vi "configureSerial.vi"(8 "error in (no error)":errorcluster, 10 "RS232Config":T1={"VISA resource name"="", "Baud Rate"=9600, "Data Bits"=8, "Parity"=enum."None", "Stop Bits"=10, "Flow Control"=0, "Timeout (ms)"=10000} {"Stop Bits" items=["1.0"=10, "1.5"=15, "2.0"=20]; "Flow Control" items=["None", "XON/XOFF", "RTS/CTS", "XON/XOFF & RTS/CTS", "DTR/DSR", "XON/XOFF & DTR/DSR"]; "Data Bits" min=5 max=8 step=1}, 11 "Model in":refnum<class "Model.lvclass">) -> (0 "error out":errorcluster, 3 "Model out":refnum<class "Model.lvclass">)   [LabVIEW 2012, in "Model.lvclass"]
uses:
  Model.lvclass
  Program Files (x86)/National Instruments/LabVIEW 2012/user.lib/Common/SerialProtocols/Configuration/RS232Config.ctl
  Program Files (x86)/National Instruments/LabVIEW 2012/user.lib/Common/SerialProtocols/Configuration/SerialProtocol.ctl
  Program Files (x86)/National Instruments/LabVIEW 2012/user.lib/Common/SerialProtocols/Implementations/SerialSimulator/SerialSimulator.lvclass
  Program Files (x86)/National Instruments/LabVIEW 2012/user.lib/Common/SerialProtocols/SerialCommunicator/SerialCommunicator.lvclass
  Model.lvclass/Model.ctl
  Program Files (x86)/National Instruments/LabVIEW 2012/user.lib/Common/SerialProtocols/Implementations/RS232/RS232.lvclass
  Program Files (x86)/National Instruments/LabVIEW 2012/user.lib/Common/SerialProtocols/Implementations/RS485/RS485.lvclass
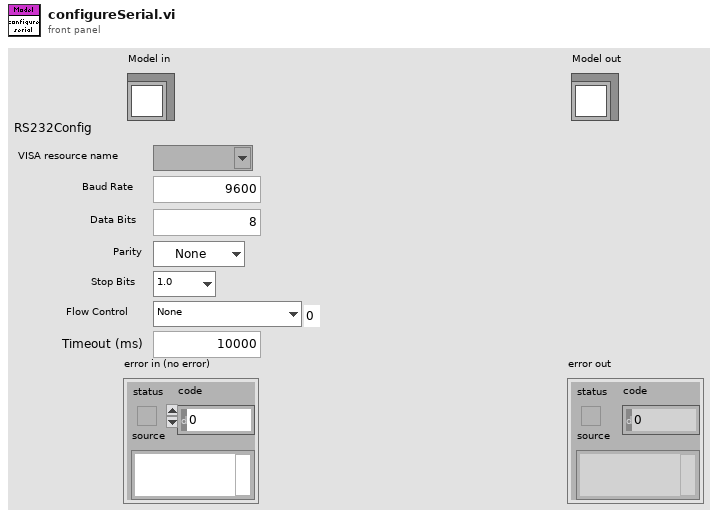
[diagram p1: front panel]
types:
  T1 = typedef "RS232Config.ctl" = cluster{"VISA resource name":refnum<visa-resource-name>, "Baud Rate":u32, "Data Bits":u16, "Parity":enum16{"None", "Odd", "Even", "Mark", "Space"}, "Stop Bits":u16, "Flow Control":u16, "Timeout (ms)":u32}
  T2 = typedef "SerialProtocol.ctl" = enum16{"RS232", "RS485", "SerialSimulator"}
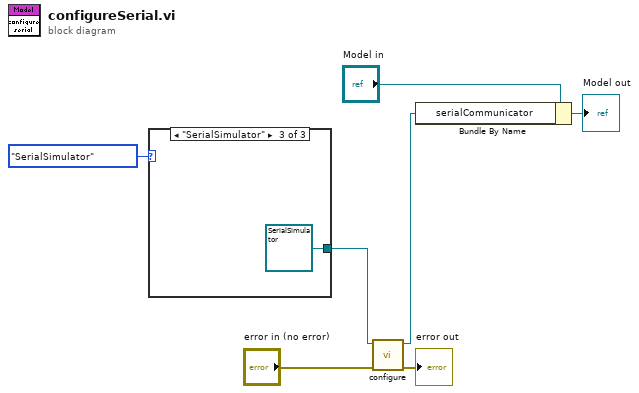
[diagram p0: block diagram]
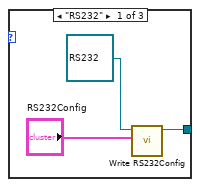
[diagram p2: hidden frame]
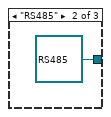
[diagram p3: hidden frame]
diagram:
  n1 = case shown="\"SerialSimulator\"" SerialProtocol."SerialSimulator" ("Serial Protocol") {
    tunnel: [w9 refnum<class "RS485.lvclass"> refnum ("RS485.lvclass") refnum<class "SerialSimulator.lvclass"> refnum ("SerialSimulator.lvclass")] -> w7
    frame "RS232" {
      n2 = call "Write RS232Config.vi"("RS232Config"="RS232Config", "RS232 in"=refnum<class "RS232.lvclass"> refnum ("RS232.lvclass")) -> ("RS232 out"=w9:refnum<class "RS232.lvclass">)  [unwired: 9 in]
    }
    frame "RS485" {
    }
    frame "SerialSimulator" {
    }
  }
  n3 = call-dynamic "configure.vi"("error in (no error)"="error in (no error)", "SerialCommunicator in"=w7) -> ("error out"=→"error out":errorcluster, "SerialCommunicator out"=w2:refnum<class "SerialCommunicator.lvclass">)  [unwired: 8 in]
  n4 = Bundle By Name(cluster="Model in", "serialCommunicator"=w2) -> (→"Model out":refnum<class "Model.lvclass">)
